vi "cps_serial_read.vi"(0 "serial in":refnum<visa-resource-name>, 8 "Range H":dbl, 9 "Range L":dbl=3.0) -> (1 "CK DATO":bool, 3 "Dato_ACK":u8, 4 "Allarme S":T1, 5 "AllarmeT":T1, 6 "CK Tot":bool, 7 "Allarme R":T1, 10 "Error Out":bool, 11 "Timeout":bool, 12 "Fase R":T3 {"Freq" format="%#.2g"; "Vout" format="%#.1f"; "Vset" format="%#.1f"}, 13 "Modo T":T2, 14 "Fase S":T3 {"Fase" format="%#.0f"; "Freq" format="%#.2g"; "Vout" format="%#.1f"; "Vset" format="%#.1f"}, 15 "Fase T":T3 {"Fase" format="%#.1f"; "Freq" format="%#.2g"; "Vout" format="%#.1f"; "Vset" format="%#.1f"}, 16 "DATI_RISP":u8[](array[numeric]), 17 "ACK":bool, 18 "Modo R":T2, 19 "Modo S":T2)   [LabVIEW 2019]
panel:
  in  "Timeout Limit":u32=3
  out "size(s)":i32
  out "Serial Read 3":string
  out "Bytes to Read":u32=10
  out "REPLY_PACKET":u8[](array[numeric])
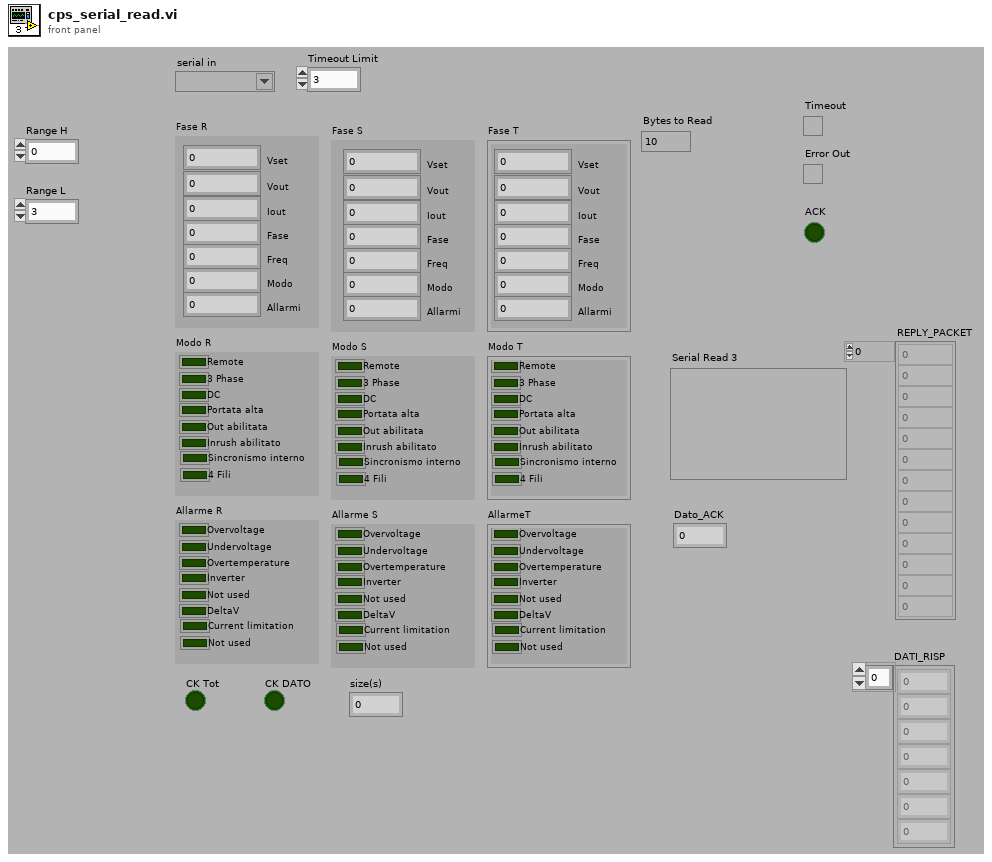
[diagram p1: front panel]
types:
  T1 = cluster{"Overvoltage":bool, "Undervoltage":bool, "Overtemperature":bool, "Inverter":bool, "Not used":bool, "DeltaV":bool, "Current limitation":bool, "Not used":bool}
  T2 = cluster{"Remote":bool, "3 Phase":bool, "DC":bool, "Portata alta":bool, "Out abilitata":bool, "Inrush abilitato":bool, "Sincronismo interno":bool, "4 Fili":bool}
  T3 = cluster{"Vset":dbl, "Vout":dbl, "Iout":dbl, "Freq":dbl, "Fase":dbl, "Modo":dbl, "Allarmi":dbl}
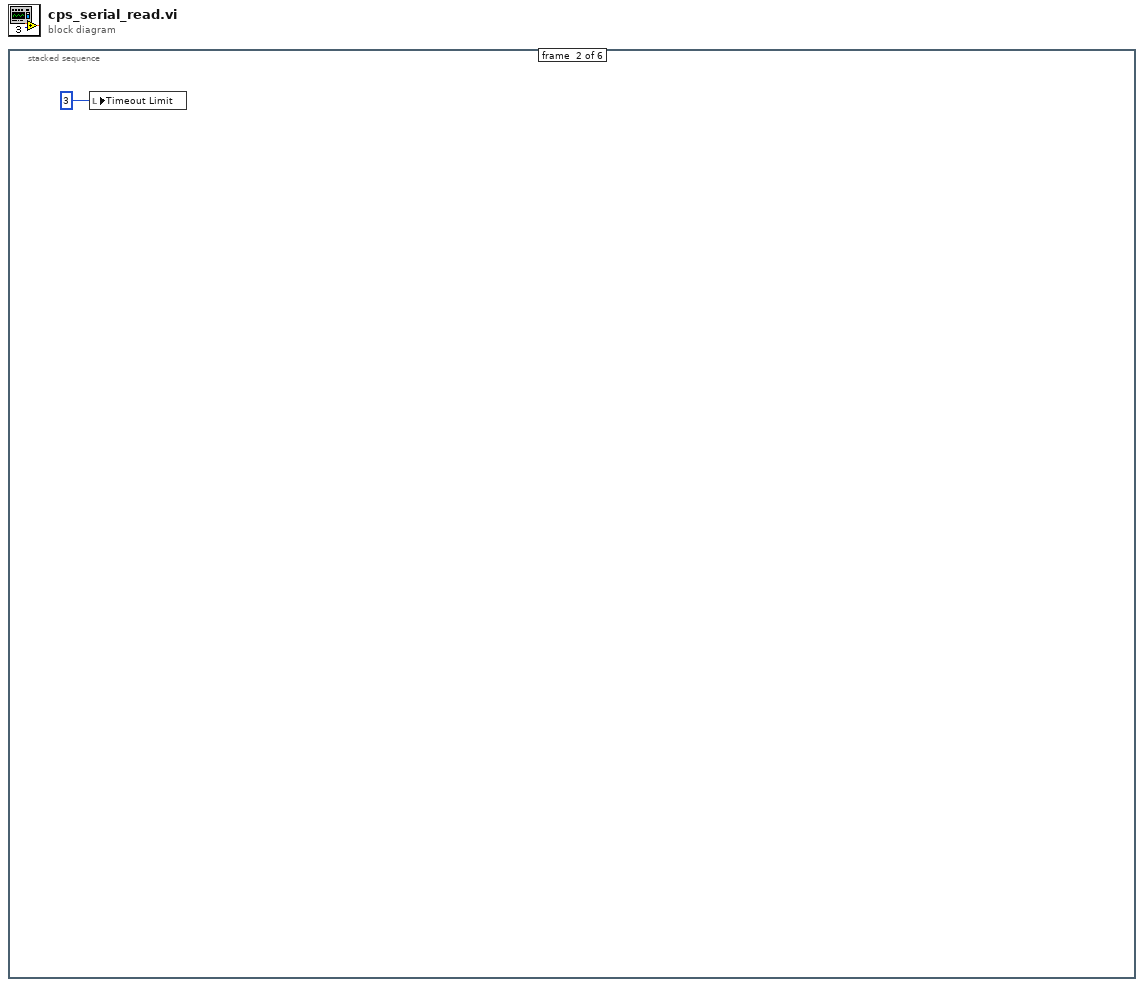
[diagram p0: block diagram]
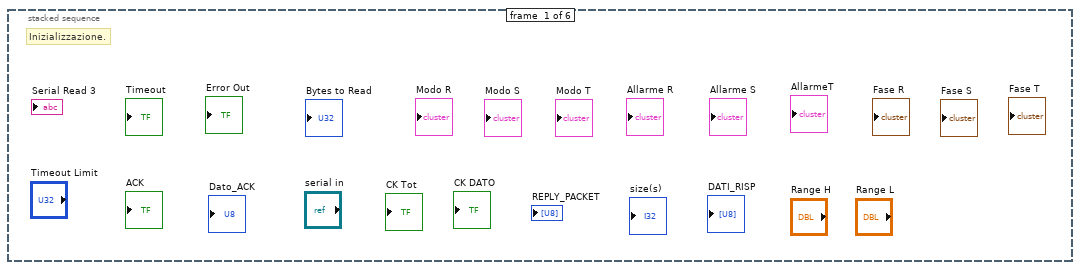
[diagram p2: hidden frame]
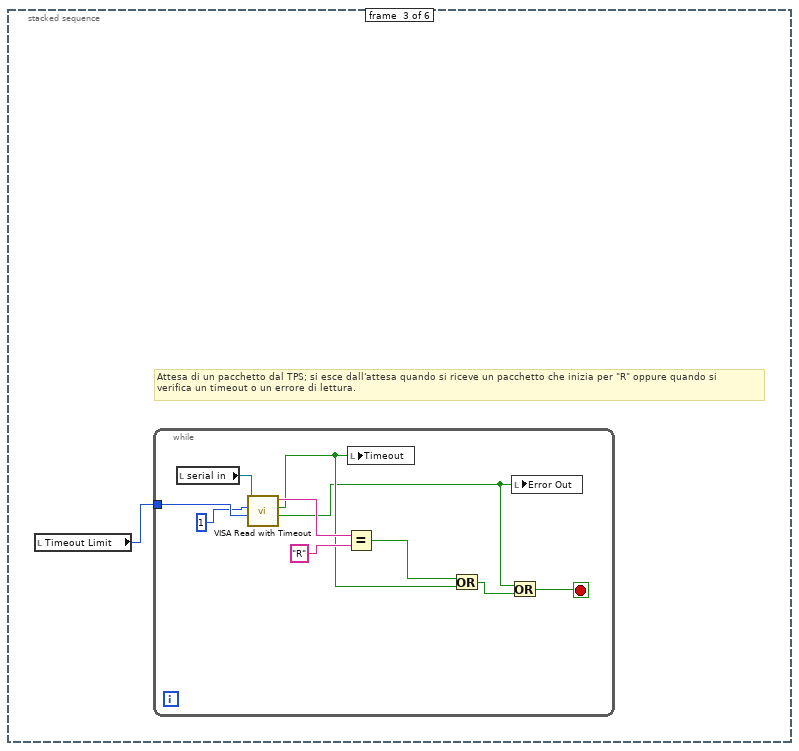
[diagram p3: hidden frame]
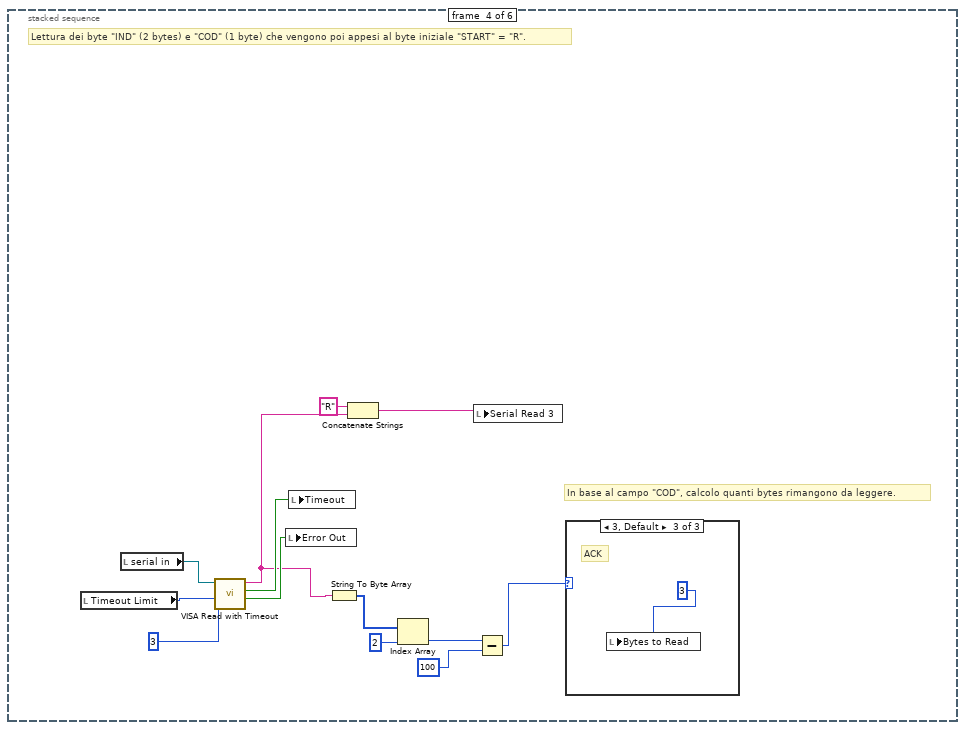
[diagram p4: hidden frame]
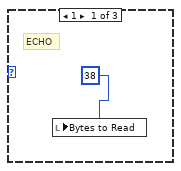
[diagram p5: hidden frame]
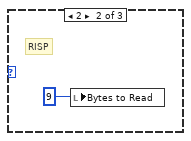
[diagram p6: hidden frame]
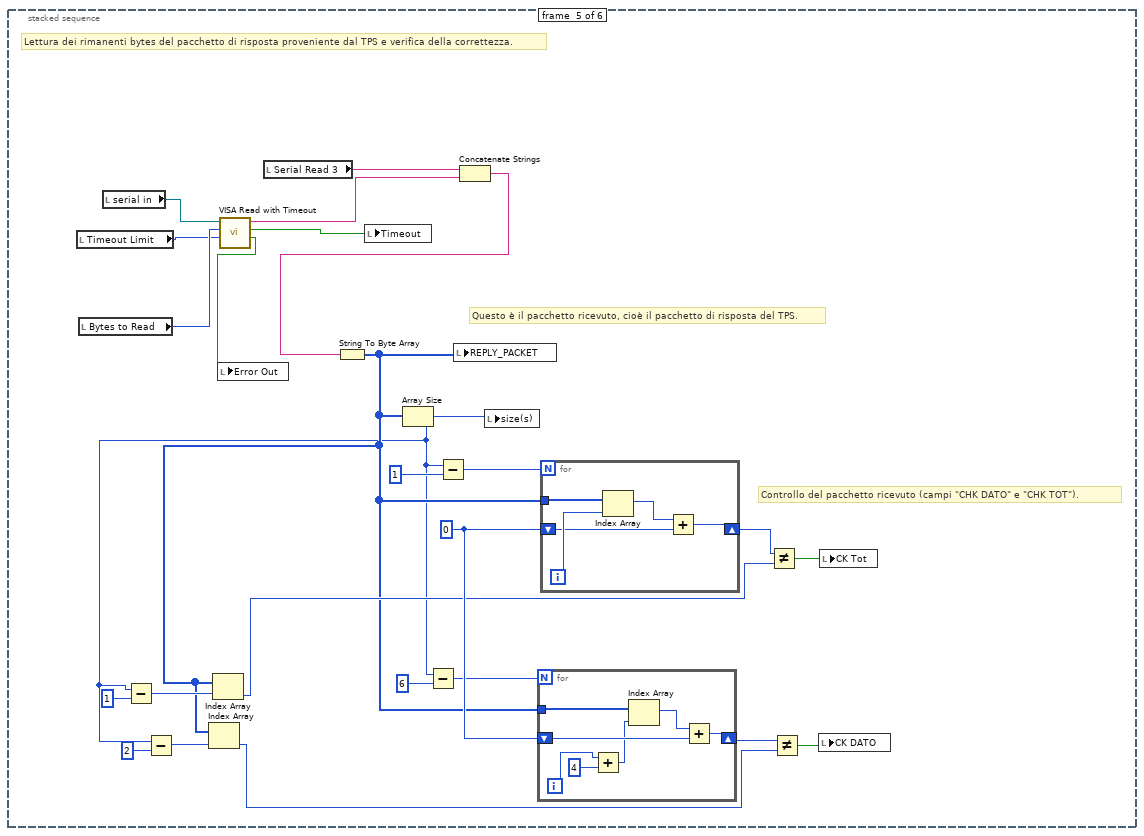
[diagram p7: hidden frame]
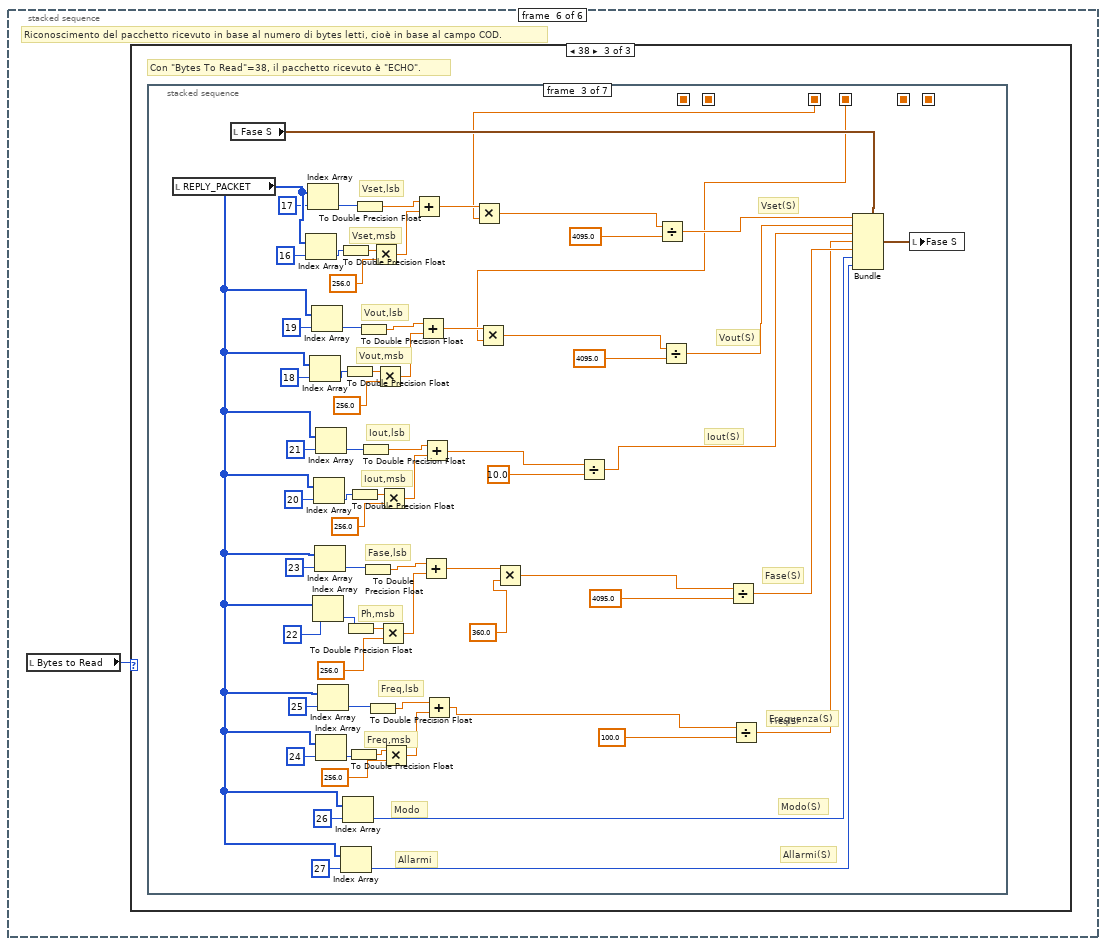
[diagram p8: hidden frame]
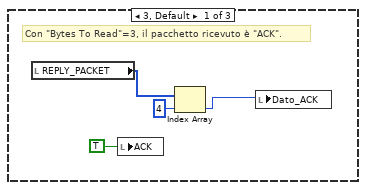
[diagram p9: hidden frame]
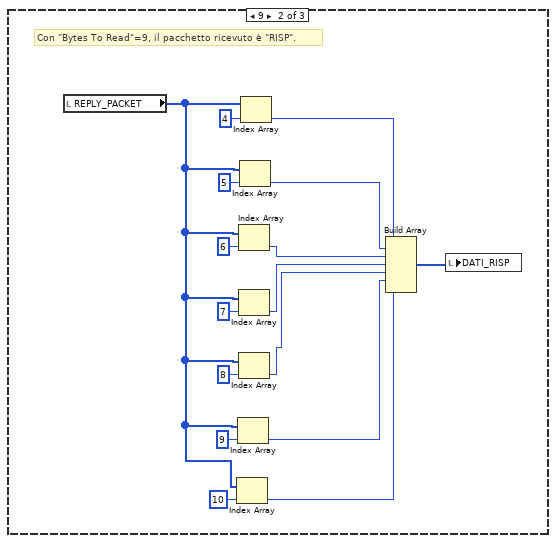
[diagram p10: hidden frame]
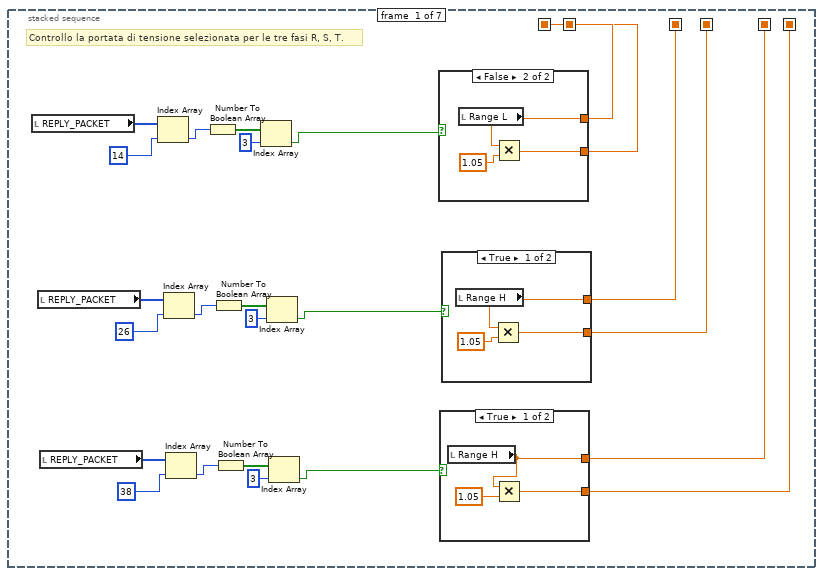
[diagram p11: hidden frame]
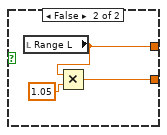
[diagram p12: hidden frame]
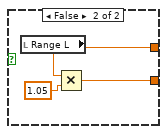
[diagram p13: hidden frame]
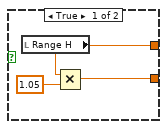
[diagram p14: hidden frame]
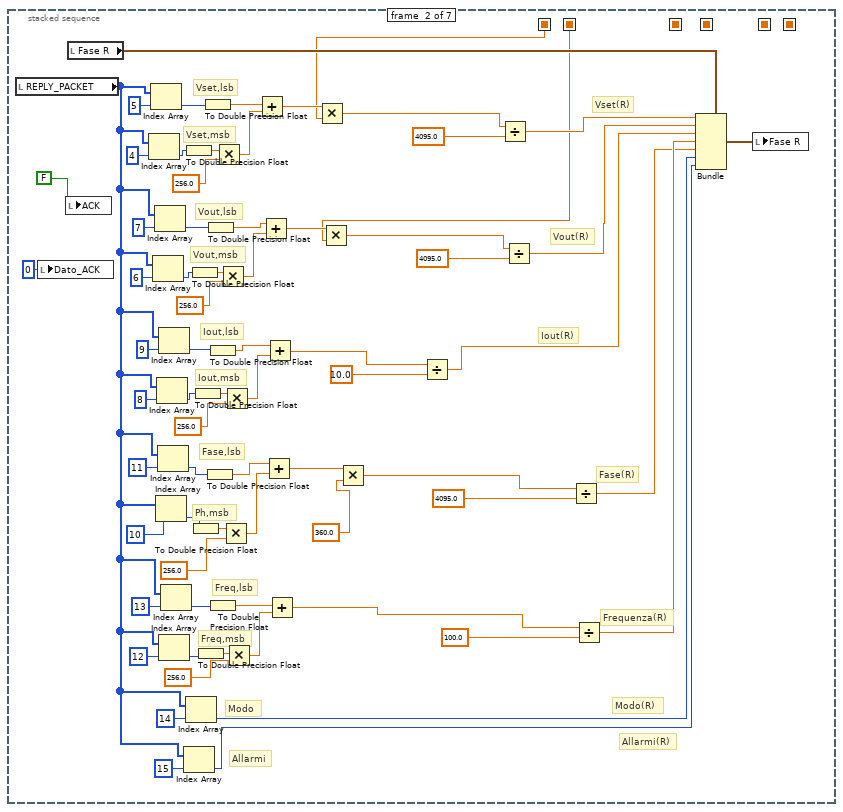
[diagram p15: hidden frame]
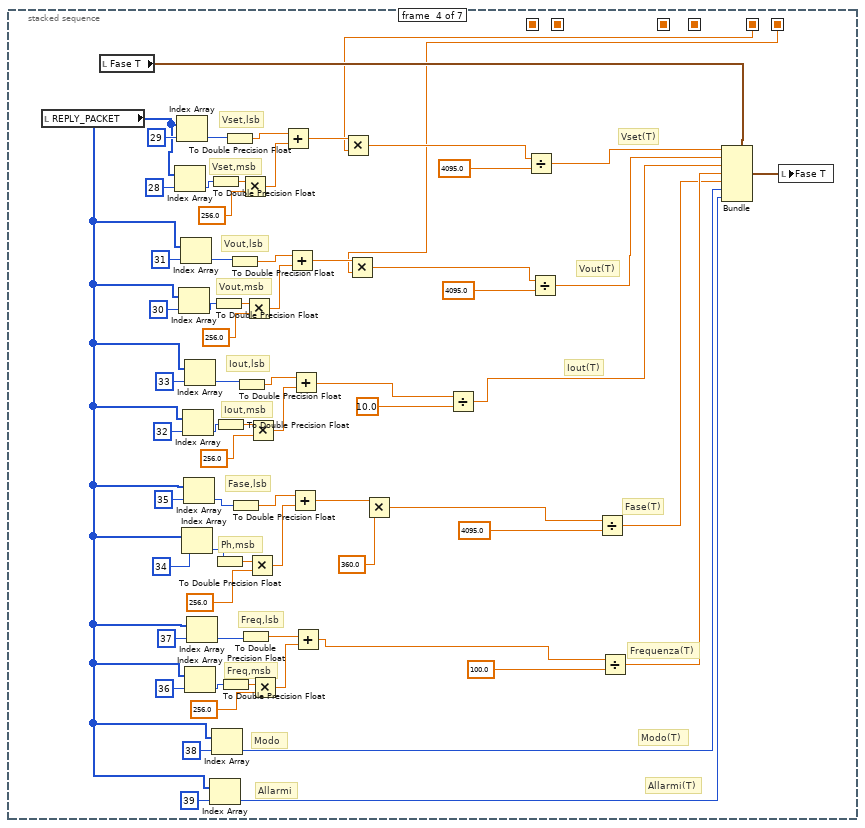
[diagram p16: hidden frame]
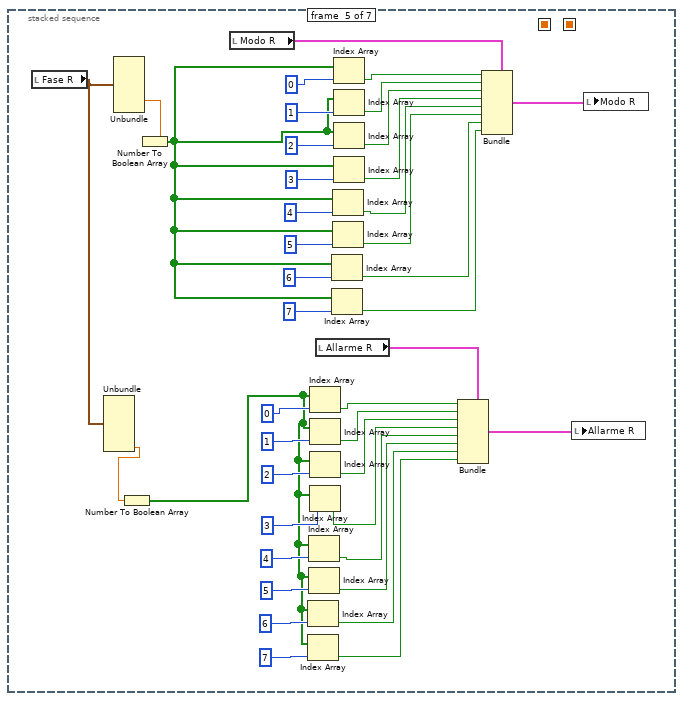
[diagram p17: hidden frame]
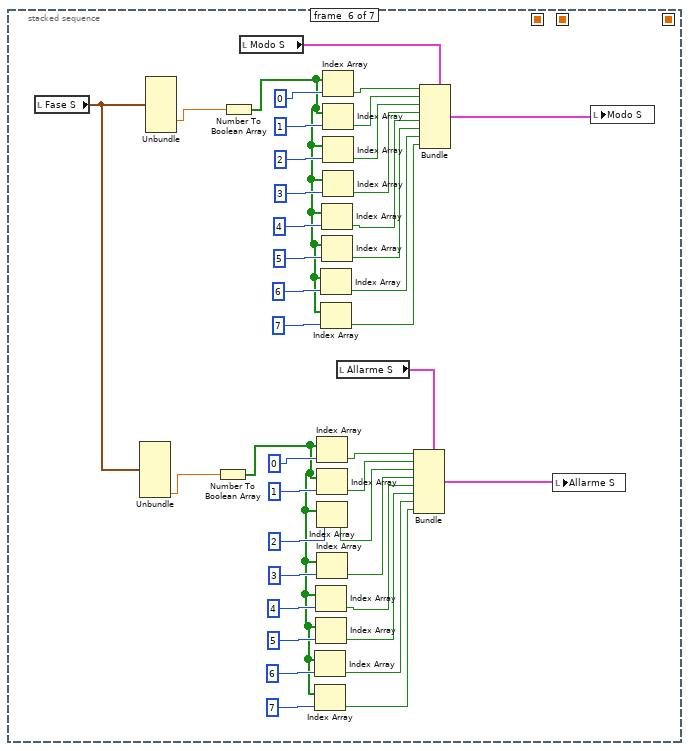
[diagram p18: hidden frame]
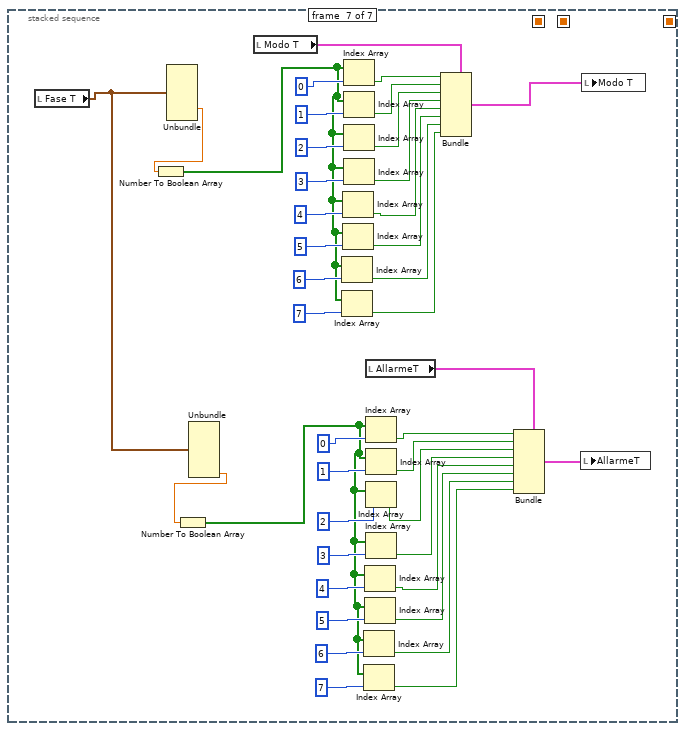
[diagram p19: hidden frame]
diagram:
  n1 = stacked-sequence {
    frame #0 {
      # "Inizializzazione."
    }
    frame #1 {
      n2 = local write "Timeout Limit"(u32 3 ("Timeout Limit")) -> ()
    }
    frame #2 {
      # "Attesa di un pacchetto dal TPS; si esce dall'attesa quando si riceve un pacchetto che inizia per \"R\" oppure quando si\nverifica un timeout o un errore di lettura."
      n3 = local read "Timeout Limit"() -> (w2:u32)
      n4 = while {
        tunnel: w2 -> [w12]
        stop <- w4 stop-if-true
        n5 = local read "serial in"() -> (w3:refnum<visa-resource-name>)
        n6 = call "VISA Read with Timeout.vi"("Timeout Limit"=w12, "Bytes to Read"=u32 1, "serial in"=w3) -> ("Error Out"=w5:bool, "Timeout"=w7:bool, "Serial Read"=w10:string)  [unwired: 1 in, 2 out]
        n7 = Equal?(x=w10, y="R") -> (x = y?=w8:bool)
        n8 = local write "Timeout"(w7) -> ()
        n9 = Or(x=w8, y=w7) -> (x .or. y?=w6:bool)
        n10 = Or(x=w5, y=w6) -> (x .or. y?=w4:bool)
        n11 = local write "Error Out"(w5) -> ()
      }
    }
    frame #3 {
      # "Lettura dei byte \"IND\" (2 bytes) e \"COD\" (1 byte) che vengono poi appesi al byte iniziale \"START\" = \"R\"."
      # "In base al campo \"COD\", calcolo quanti bytes rimangono da leggere."
      n12 = local read "Timeout Limit"() -> (w14:u32)
      n13 = local read "serial in"() -> (w13:refnum<visa-resource-name>)
      n14 = call "VISA Read with Timeout.vi"("Timeout Limit"=w14, "Bytes to Read"=u32 3, "serial in"=w13) -> ("Error Out"=w23:bool, "Timeout"=w24:bool, "Serial Read"=w20:string)  [unwired: 1 in, 2 out]
      n15 = local write "Error Out"(w23) -> ()
      n16 = local write "Timeout"(w24) -> ()
      n17 = String To Byte Array(string=w20) -> (unsigned byte array=w19:u8[])
      n18 = Concatenate Strings "Concatenate Strings"("R" ("string"), w20) -> (w21:string)
      n19 = Index Array "Index Array"(array=w19, index=2) -> (element=w17:u8)
      n20 = local write "Serial Read 3"(w21) -> ()
      n21 = Subtract(x=w17, y=u32 100 ("Bytes to Read")) -> (x-y=w16:u32)
      n22 = case shown="3, Default" w16 {
        frame 1 {
          # "ECHO"
          n23 = local write "Bytes to Read"(38 ("index")) -> ()
        }
        frame 2 {
          # "RISP"
          n24 = local write "Bytes to Read"(9 ("index")) -> ()
        }
        frame 3, Default {
          # "ACK"
          n25 = local write "Bytes to Read"(u32 3 ("Bytes to Read")) -> ()
        }
      }
    }
    frame #4 {
      w46 = u8 0
      # "Controllo del pacchetto ricevuto (campi \"CHK DATO\" e \"CHK TOT\")."
      # "Questo è il pacchetto ricevuto, cioè il pacchetto di risposta del TPS."
      # "Lettura dei rimanenti bytes del pacchetto di risposta proveniente dal TPS e verifica della correttezza."
      n26 = local read "Timeout Limit"() -> (w34:u32)
      n27 = local read "Bytes to Read"() -> (w43:u32)
      n28 = local read "serial in"() -> (w33:refnum<visa-resource-name>)
      n29 = call "VISA Read with Timeout.vi"("Timeout Limit"=w34, "Bytes to Read"=w43, "serial in"=w33) -> ("Error Out"=w53:bool, "Timeout"=w52:bool, "Serial Read"=w51:string)  [unwired: 1 in, 2 out]
      n30 = local write "Error Out"(w53) -> ()
      n31 = local read "Serial Read 3"() -> (w49:string)
      n32 = local write "Timeout"(w52) -> ()
      n33 = Concatenate Strings "Concatenate Strings"(w49, w51) -> (w50:string)
      n34 = String To Byte Array(string=w50) -> (unsigned byte array=w30:u8[])
      n35 = Array Size(array=w30) -> (size(s)=w29:i32)
      n36 = Subtract(x=w29, y=1) -> (x-y=w42:i32)
      n37 = Subtract(x=w29, y=2) -> (x-y=w41:i32)
      n38 = Index Array "Index Array"(array=w30, index=w41) -> (element=w35:u8)
      n39 = Index Array "Index Array"(array=w30, index=w42) -> (element=w37:u8)
      n40 = Subtract(x=w29, y=u8 6) -> (x-y=w45:i32)
      n41 = Subtract(x=w29, y=u8 1) -> (x-y=w47:i32)
      n42 = local write "REPLY_PACKET"(w30) -> ()
      n43 = local write "size(s)"(w29) -> ()
      n44 = for {
        N: w45 -> [_]
        tunnel: w30 -> [w60]
        shift-right: [w57] -> w36
        shift-left: w46 -> [w58]
        i -> [w55]
        n45 = Add(x=w55, y=u32 4) -> (x+y=w54:u32)
        n46 = Index Array(array=w60, index=w54) -> (element=w59:u8)
        n47 = Add(x=w59, y=w58) -> (x+y=w57:u8)
      }
      n48 = for {
        N: w47 -> [_]
        tunnel: w30 -> [w65]
        shift-right: [w61] -> w38
        shift-left: w46 -> [w62]
        i -> [w63]
        n49 = Index Array "Index Array"(array=w65, index=w63) -> (element=w64:u8)
        n50 = Add(x=w64, y=w62) -> (x+y=w61:u8)
      }
      n51 = Not Equal?(x=w38, y=w37) -> (x != y?=w32:bool)
      n52 = Not Equal?(x=w36, y=w35) -> (x != y?=w31:bool)
      n53 = local write "CK DATO"(w31) -> ()
      n54 = local write "CK Tot"(w32) -> ()
    }
    frame #5 {
      # "Riconoscimento del pacchetto ricevuto in base al numero di bytes letti, cioè in base al campo COD."
      n55 = local read "Bytes to Read"() -> (w66:u32)
      n56 = case shown="38" w66 {
        frame 3, Default {
          # "Con \"Bytes To Read\"=3, il pacchetto ricevuto è \"ACK\"."
          n57 = local read "REPLY_PACKET"() -> (w70:u8[])
          n58 = local write "ACK"(TRUE ("ACK")) -> ()
          n59 = Index Array "Index Array"(array=w70, index=4) -> (element=w67:u8)
          n60 = local write "Dato_ACK"(w67) -> ()
        }
        frame 9 {
          # "Con \"Bytes To Read\"=9, il pacchetto ricevuto è \"RISP\"."
          n61 = local read "REPLY_PACKET"() -> (w79:u8[])
          n62 = Index Array "Index Array"(array=w79, index=10) -> (element=w72:u8)
          n63 = Index Array "Index Array"(array=w79, index=9) -> (element=w73:u8)
          n64 = Index Array "Index Array"(array=w79, index=6) -> (element=w76:u8)
          n65 = Index Array "Index Array"(array=w79, index=7) -> (element=w75:u8)
          n66 = Index Array "Index Array"(array=w79, index=8) -> (element=w74:u8)
          n67 = Index Array "Index Array"(array=w79, index=5) -> (element=w77:u8)
          n68 = Index Array "Index Array"(array=w79, index=4) -> (element=w78:u8)
          n69 = Build Array(w78, w77, w76, w75, w74, w73, w72) -> (w71:u8[])
          n70 = local write "DATI_RISP"(w71) -> ()
        }
        frame 38 {
          # "Con \"Bytes To Read\"=38, il pacchetto ricevuto è \"ECHO\"."
          n71 = stacked-sequence {
            seq-local: [w110 _ _ _ _ _ _] -> [_ w150 _ _ _ _ _]
            seq-local: [w109 _ _ _ _ _ _] -> [_ w149 _ _ _ _ _]
            seq-local: [w108 _ _ _ _ _ _] -> [_ _ w220 _ _ _ _]
            seq-local: [w107 _ _ _ _ _ _] -> [_ _ w219 _ _ _ _]
            seq-local: [w106 _ _ _ _ _ _] -> [_ _ _ w288 _ _ _]
            seq-local: [w105 _ _ _ _ _ _] -> [_ _ _ w287 _ _ _]
            frame #0 {
              # "Controllo la portata di tensione selezionata per le tre fasi R, S, T."
              n72 = local read "REPLY_PACKET"() -> (w104:u8[])
              n73 = local read "REPLY_PACKET"() -> (w94:u8[])
              n74 = local read "REPLY_PACKET"() -> (w92:u8[])
              n75 = Index Array "Index Array"(array=w104, index=14) -> (element=w102:u8)
              n76 = Index Array "Index Array"(array=w94, index=26) -> (element=w96:u8)
              n77 = Index Array "Index Array"(array=w92, index=38) -> (element=w90:u8)
              n78 = Number To Boolean Array(number=w102) -> (Boolean array=w101:bool[])
              n79 = Number To Boolean Array(number=w96) -> (Boolean array=w97:bool[])
              n80 = Number To Boolean Array(number=w90) -> (Boolean array=w89:bool[])
              n81 = Index Array "Index Array"(array=w101, index=3) -> (element=w99:bool)
              n82 = Index Array "Index Array"(array=w97, index=3) -> (element=w93:bool)
              n83 = Index Array "Index Array"(array=w89, index=3) -> (element=w87:bool)
              n84 = case shown="False" w99 {
                tunnel: [w125 w127] -> w110
                tunnel: [w123 w128] -> w109
                frame True {
                  n85 = local read "Range H"() -> (w125:dbl)
                  n86 = Multiply(x=w125, y=1.05) -> (x*y=w123:dbl)
                }
                frame False {
                  n87 = local read "Range L"() -> (w127:dbl)
                  n88 = Multiply(x=w127, y=1.05) -> (x*y=w128:dbl)
                }
              }
              n89 = case shown="True" w87 {
                tunnel: [w112 w115] -> w106
                tunnel: [w113 w116] -> w105
                frame True {
                  n90 = local read "Range H"() -> (w112:dbl)
                  n91 = Multiply(x=w112, y=1.05) -> (x*y=w113:dbl)
                }
                frame False {
                  n92 = local read "Range L"() -> (w115:dbl)
                  n93 = Multiply(x=w115, y=1.05) -> (x*y=w116:dbl)
                }
              }
              n94 = case shown="True" w93 {
                tunnel: [w118 w121] -> w108
                tunnel: [w119 w122] -> w107
                frame True {
                  n95 = local read "Range H"() -> (w118:dbl)
                  n96 = Multiply(x=w118, y=1.05) -> (x*y=w119:dbl)
                }
                frame False {
                  n97 = local read "Range L"() -> (w121:dbl)
                  n98 = Multiply(x=w121, y=1.05) -> (x*y=w122:dbl)
                }
              }
            }
            frame #1 {
              # "Allarmi(R)"
              # "Modo(R)"
              # "Frequenza(R)"
              # "Fase(R)"
              # "Iout(R)"
              # "Vout(R)"
              # "Vset(R)"
              # "Allarmi"
              # "Modo"
              # "Freq,msb"
              # "Freq,lsb"
              # "Ph,msb"
              # "Fase,lsb"
              # "Iout,msb"
              # "Iout,lsb"
              # "Vout,msb"
              # "Vout,lsb"
              # "Vset,lsb"
              # "Vset,msb"
              n99 = local read "REPLY_PACKET"() -> (w153:u8[])
              n100 = local write "Dato_ACK"(u8 0 ("Dato_ACK")) -> ()
              n101 = local write "ACK"(FALSE ("ACK")) -> ()
              n102 = local read "Fase R"() -> (w184:T3)
              n103 = Index Array(array=w153, index=4) -> (element=w136:u8)
              n104 = Index Array "Index Array"(array=w153, index=5) -> (element=w148:u8)
              n105 = Index Array(array=w153, index=6) -> (element=w138:u8)
              n106 = Index Array(array=w153, index=7) -> (element=w146:u8)
              n107 = Index Array(array=w153, index=10) -> (element=w134:u8)
              n108 = Index Array(array=w153, index=8) -> (element=w140:u8)
              n109 = Index Array(array=w153, index=11) -> (element=w142:u8)
              n110 = Index Array(array=w153, index=9) -> (element=w144:u8)
              n111 = Index Array(array=w153, index=12) -> (element=w130:u8)
              n112 = Index Array(array=w153, index=13) -> (element=w132:u8)
              n113 = To Double Precision Float(number=w136) -> (double precision float=w135:dbl)
              n114 = Index Array(array=w153, index=15) -> (element=w155:u8)
              n115 = Index Array(array=w153, index=14) -> (element=w156:u8)
              n116 = To Double Precision Float(number=w138) -> (double precision float=w137:dbl)
              n117 = To Double Precision Float(number=w134) -> (double precision float=w133:dbl)
              n118 = To Double Precision Float(number=w140) -> (double precision float=w139:dbl)
              n119 = To Double Precision Float(number=w130) -> (double precision float=w129:dbl)
              n120 = To Double Precision Float(number=w148) -> (double precision float=w147:dbl)
              n121 = To Double Precision Float(number=w142) -> (double precision float=w141:dbl)
              n122 = To Double Precision Float(number=w146) -> (double precision float=w145:dbl)
              n123 = To Double Precision Float(number=w144) -> (double precision float=w143:dbl)
              n124 = To Double Precision Float(number=w132) -> (double precision float=w131:dbl)
              n125 = Multiply(x=w135, y=256.0) -> (x*y=w194:dbl)
              n126 = Multiply(x=w137, y=256.0) -> (x*y=w187:dbl)
              n127 = Multiply(x=w133, y=256.0) -> (x*y=w170:dbl)
              n128 = Multiply(x=w139, y=256.0) -> (x*y=w177:dbl)
              n129 = Multiply(x=w129, y=256.0) -> (x*y=w162:dbl)
              n130 = Add(x=w147, y=w194) -> (x+y=w193:dbl)
              n131 = Add(x=w145, y=w187) -> (x+y=w186:dbl)
              n132 = Add(x=w141, y=w170) -> (x+y=w166:dbl)
              n133 = Add(x=w143, y=w177) -> (x+y=w175:dbl)
              n134 = Add(x=w131, y=w162) -> (x+y=w154:dbl)
              n135 = Multiply(x=w193, y=w150) -> (x*y=w192:dbl)
              n136 = Multiply(x=w186, y=w149) -> (x*y=w185:dbl)
              n137 = Multiply(x=w166, y=360.0) -> (x*y=w167:dbl)
              n138 = Divide(x=w175, y=10.0) -> (x/y=w174:dbl)
              n139 = Divide(x=w192, y=4095.0) -> (x/y=w183:dbl)
              n140 = Divide(x=w185, y=4095.0) -> (x/y=w181:dbl)
              n141 = Divide(x=w167, y=4095.0) -> (x/y=w159:dbl)
              n142 = Divide(x=w154, y=100.0) -> (x/y=w160:dbl)
              n143 = Bundle "Bundle"(cluster=w184, "Vset"=w183, "Vout"=w181, "Iout"=w174, "Freq"=w160, "Fase"=w159, "Modo"=w156, "Allarmi"=w155) -> (w182:T3)
              n144 = local write "Fase R"(w182) -> ()
            }
            frame #2 {
              # "Allarmi(S)"
              # "Modo(S)"
              # "Frequenza(S)"
              # "Fase(S)"
              # "Iout(S)"
              # "Vout(S)"
              # "Vset(S)"
              # "Allarmi"
              # "Modo"
              # "Freq,msb"
              # "Freq,lsb"
              # "Ph,msb"
              # "Fase,lsb"
              # "Iout,msb"
              # "Iout,lsb"
              # "Vout,msb"
              # "Vout,lsb"
              # "Vset,lsb"
              # "Vset,msb"
              # "Freq(S)"
              n145 = local read "REPLY_PACKET"() -> (w263:u8[])
              n146 = local read "Fase S"() -> (w235:T3)
              n147 = Index Array(array=w263, index=16) -> (element=w216:u8)
              n148 = Index Array(array=w263, index=17) -> (element=w218:u8)
              n149 = Index Array(array=w263, index=18) -> (element=w212:u8)
              n150 = Index Array(array=w263, index=19) -> (element=w214:u8)
              n151 = Index Array(array=w263, index=22) -> (element=w204:u8)
              n152 = Index Array(array=w263, index=20) -> (element=w208:u8)
              n153 = Index Array(array=w263, index=23) -> (element=w206:u8)
              n154 = Index Array(array=w263, index=21) -> (element=w210:u8)
              n155 = Index Array(array=w263, index=24) -> (element=w200:u8)
              n156 = Index Array(array=w263, index=25) -> (element=w202:u8)
              n157 = To Double Precision Float(number=w216) -> (double precision float=w215:dbl)
              n158 = Index Array(array=w263, index=27) -> (element=w265:u8)
              n159 = Index Array(array=w263, index=26) -> (element=w264:u8)
              n160 = To Double Precision Float(number=w212) -> (double precision float=w211:dbl)
              n161 = To Double Precision Float(number=w204) -> (double precision float=w203:dbl)
              n162 = To Double Precision Float(number=w200) -> (double precision float=w199:dbl)
              n163 = To Double Precision Float(number=w208) -> (double precision float=w207:dbl)
              n164 = To Double Precision Float(number=w218) -> (double precision float=w217:dbl)
              n165 = To Double Precision Float(number=w214) -> (double precision float=w213:dbl)
              n166 = To Double Precision Float(number=w210) -> (double precision float=w209:dbl)
              n167 = To Double Precision Float(number=w206) -> (double precision float=w205:dbl)
              n168 = To Double Precision Float(number=w202) -> (double precision float=w201:dbl)
              n169 = Multiply(x=w215, y=256.0) -> (x*y=w225:dbl)
              n170 = Multiply(x=w211, y=256.0) -> (x*y=w232:dbl)
              n171 = Multiply(x=w203, y=256.0) -> (x*y=w249:dbl)
              n172 = Multiply(x=w207, y=256.0) -> (x*y=w242:dbl)
              n173 = Multiply(x=w199, y=256.0) -> (x*y=w257:dbl)
              n174 = Add(x=w217, y=w225) -> (x+y=w226:dbl)
              n175 = Add(x=w213, y=w232) -> (x+y=w233:dbl)
              n176 = Add(x=w205, y=w249) -> (x+y=w253:dbl)
              n177 = Add(x=w209, y=w242) -> (x+y=w244:dbl)
              n178 = Add(x=w201, y=w257) -> (x+y=w266:dbl)
              n179 = Multiply(x=w226, y=w220) -> (x*y=w227:dbl)
              n180 = Multiply(x=w233, y=w219) -> (x*y=w234:dbl)
              n181 = Multiply(x=w253, y=360.0) -> (x*y=w252:dbl)
              n182 = Divide(x=w244, y=10.0) -> (x/y=w245:dbl)
              n183 = Divide(x=w227, y=4095.0) -> (x/y=w236:dbl)
              n184 = Divide(x=w234, y=4095.0) -> (x/y=w238:dbl)
              n185 = Divide(x=w252, y=4095.0) -> (x/y=w260:dbl)
              n186 = Divide(x=w266, y=100.0) -> (x/y=w259:dbl)
              n187 = Bundle "Bundle"(cluster=w235, "Vset"=w236, "Vout"=w238, "Iout"=w245, "Freq"=w259, "Fase"=w260, "Modo"=w264, "Allarmi"=w265) -> (w237:T3)
              n188 = local write "Fase S"(w237) -> ()
            }
            frame #3 {
              # "Allarmi(T)"
              # "Modo(T)"
              # "Frequenza(T)"
              # "Fase(T)"
              # "Iout(T)"
              # "Vout(T)"
              # "Vset(T)"
              # "Allarmi"
              # "Modo"
              # "Freq,msb"
              # "Freq,lsb"
              # "Ph,msb"
              # "Fase,lsb"
              # "Iout,msb"
              # "Iout,lsb"
              # "Vout,msb"
              # "Vout,lsb"
              # "Vset,lsb"
              # "Vset,msb"
              n189 = local read "REPLY_PACKET"() -> (w292:u8[])
              n190 = local read "Fase T"() -> (w320:T3)
              n191 = Index Array(array=w292, index=28) -> (element=w284:u8)
              n192 = Index Array(array=w292, index=29) -> (element=w286:u8)
              n193 = Index Array(array=w292, index=30) -> (element=w280:u8)
              n194 = Index Array(array=w292, index=31) -> (element=w282:u8)
              n195 = Index Array(array=w292, index=34) -> (element=w272:u8)
              n196 = Index Array(array=w292, index=32) -> (element=w276:u8)
              n197 = Index Array(array=w292, index=35) -> (element=w274:u8)
              n198 = Index Array(array=w292, index=33) -> (element=w278:u8)
              n199 = Index Array(array=w292, index=36) -> (element=w268:u8)
              n200 = Index Array(array=w292, index=37) -> (element=w270:u8)
              n201 = Index Array(array=w292, index=39) -> (element=w290:u8)
              n202 = To Double Precision Float(number=w284) -> (double precision float=w283:dbl)
              n203 = Index Array(array=w292, index=38) -> (element=w291:u8)
              n204 = To Double Precision Float(number=w280) -> (double precision float=w279:dbl)
              n205 = To Double Precision Float(number=w272) -> (double precision float=w271:dbl)
              n206 = To Double Precision Float(number=w276) -> (double precision float=w275:dbl)
              n207 = To Double Precision Float(number=w268) -> (double precision float=w267:dbl)
              n208 = To Double Precision Float(number=w286) -> (double precision float=w285:dbl)
              n209 = To Double Precision Float(number=w282) -> (double precision float=w281:dbl)
              n210 = To Double Precision Float(number=w274) -> (double precision float=w273:dbl)
              n211 = To Double Precision Float(number=w278) -> (double precision float=w277:dbl)
              n212 = Multiply(x=w283, y=256.0) -> (x*y=w330:dbl)
              n213 = To Double Precision Float(number=w270) -> (double precision float=w269:dbl)
              n214 = Multiply(x=w279, y=256.0) -> (x*y=w323:dbl)
              n215 = Multiply(x=w271, y=256.0) -> (x*y=w306:dbl)
              n216 = Multiply(x=w275, y=256.0) -> (x*y=w313:dbl)
              n217 = Multiply(x=w267, y=256.0) -> (x*y=w298:dbl)
              n218 = Add(x=w285, y=w330) -> (x+y=w329:dbl)
              n219 = Add(x=w281, y=w323) -> (x+y=w322:dbl)
              n220 = Add(x=w273, y=w306) -> (x+y=w302:dbl)
              n221 = Add(x=w277, y=w313) -> (x+y=w311:dbl)
              n222 = Add(x=w269, y=w298) -> (x+y=w289:dbl)
              n223 = Multiply(x=w329, y=w288) -> (x*y=w328:dbl)
              n224 = Multiply(x=w322, y=w287) -> (x*y=w321:dbl)
              n225 = Multiply(x=w302, y=360.0) -> (x*y=w303:dbl)
              n226 = Divide(x=w311, y=10.0) -> (x/y=w310:dbl)
              n227 = Divide(x=w328, y=4095.0) -> (x/y=w319:dbl)
              n228 = Divide(x=w321, y=4095.0) -> (x/y=w317:dbl)
              n229 = Divide(x=w303, y=4095.0) -> (x/y=w295:dbl)
              n230 = Divide(x=w289, y=100.0) -> (x/y=w296:dbl)
              n231 = Bundle "Bundle"(cluster=w320, "Vset"=w319, "Vout"=w317, "Iout"=w310, "Freq"=w296, "Fase"=w295, "Modo"=w291, "Allarmi"=w290) -> (w318:T3)
              n232 = local write "Fase T"(w318) -> ()
            }
            frame #4 {
              n233 = local read "Fase R"() -> (w339:T3)
              n234 = Unbundle "Unbundle"(w339) -> ("Allarmi"=w335:dbl)  [unwired: 6 out]
              n235 = Unbundle "Unbundle"(w339) -> ("Modo"=w336:dbl)  [unwired: 6 out]
              n236 = Number To Boolean Array(number=w335) -> (Boolean array=w348:bool[])
              n237 = Number To Boolean Array(number=w336) -> (Boolean array=w366:bool[])
              n238 = local read "Modo R"() -> (w375:T2)
              n239 = Index Array(array=w348, index=6) -> (element=w345:bool)
              n240 = Index Array(array=w348, index=7) -> (element=w346:bool)
              n241 = Index Array(array=w348, index=4) -> (element=w343:bool)
              n242 = Index Array(array=w348, index=5) -> (element=w344:bool)
              n243 = Index Array "Index Array"(array=w348, index=0) -> (element=w347:bool)
              n244 = Index Array(array=w348, index=1) -> (element=w340:bool)
              n245 = Index Array(array=w348, index=2) -> (element=w341:bool)
              n246 = Index Array(array=w348, index=3) -> (element=w342:bool)
              n247 = local read "Allarme R"() -> (w338:T1)
              n248 = Index Array(array=w366, index=6) -> (element=w363:bool)
              n249 = Index Array(array=w366, index=7) -> (element=w364:bool)
              n250 = Index Array(array=w366, index=4) -> (element=w361:bool)
              n251 = Index Array(array=w366, index=5) -> (element=w362:bool)
              n252 = Index Array "Index Array"(array=w366, index=0) -> (element=w365:bool)
              n253 = Index Array(array=w366, index=1) -> (element=w358:bool)
              n254 = Index Array(array=w366, index=2) -> (element=w359:bool)
              n255 = Index Array(array=w366, index=3) -> (element=w360:bool)
              n256 = Bundle(cluster=w338, "Overvoltage"=w347, "Undervoltage"=w340, "Overtemperature"=w341, "Inverter"=w342, "Not used"=w343, "DeltaV"=w344, "Current limitation"=w345, "Not used"=w346) -> (w337:T1)
              n257 = Bundle "Bundle"(cluster=w375, "Remote"=w365, "3 Phase"=w358, "DC"=w359, "Portata alta"=w360, "Out abilitata"=w361, "Inrush abilitato"=w362, "Sincronismo interno"=w363, "4 Fili"=w364) -> (w357:T2)
              n258 = local write "Allarme R"(w337) -> ()
              n259 = local write "Modo R"(w357) -> ()
            }
            frame #5 {
              n260 = local read "Fase S"() -> (w380:T3)
              n261 = Unbundle(w380) -> ("Allarmi"=w376:dbl)  [unwired: 6 out]
              n262 = Unbundle "Unbundle"(w380) -> ("Modo"=w377:dbl)  [unwired: 6 out]
              n263 = Number To Boolean Array(number=w376) -> (Boolean array=w389:bool[])
              n264 = Number To Boolean Array(number=w377) -> (Boolean array=w408:bool[])
              n265 = local read "Modo S"() -> (w399:T2)
              n266 = Index Array(array=w389, index=6) -> (element=w386:bool)
              n267 = Index Array(array=w389, index=7) -> (element=w387:bool)
              n268 = Index Array(array=w389, index=4) -> (element=w384:bool)
              n269 = Index Array(array=w389, index=5) -> (element=w385:bool)
              n270 = Index Array "Index Array"(array=w389, index=0) -> (element=w388:bool)
              n271 = Index Array(array=w389, index=1) -> (element=w381:bool)
              n272 = Index Array(array=w389, index=2) -> (element=w382:bool)
              n273 = Index Array(array=w389, index=3) -> (element=w383:bool)
              n274 = Index Array(array=w408, index=6) -> (element=w405:bool)
              n275 = Index Array(array=w408, index=7) -> (element=w406:bool)
              n276 = Index Array(array=w408, index=4) -> (element=w403:bool)
              n277 = Index Array(array=w408, index=5) -> (element=w404:bool)
              n278 = Index Array "Index Array"(array=w408, index=0) -> (element=w407:bool)
              n279 = Index Array(array=w408, index=1) -> (element=w400:bool)
              n280 = Index Array(array=w408, index=2) -> (element=w401:bool)
              n281 = Index Array(array=w408, index=3) -> (element=w402:bool)
              n282 = local read "Allarme S"() -> (w379:T1)
              n283 = Bundle(cluster=w379, "Overvoltage"=w388, "Undervoltage"=w381, "Overtemperature"=w382, "Inverter"=w383, "Not used"=w384, "DeltaV"=w385, "Current limitation"=w386, "Not used"=w387) -> (w378:T1)
              n284 = Bundle(cluster=w399, "Remote"=w407, "3 Phase"=w400, "DC"=w401, "Portata alta"=w402, "Out abilitata"=w403, "Inrush abilitato"=w404, "Sincronismo interno"=w405, "4 Fili"=w406) -> (w398:T2)
              n285 = local write "Allarme S"(w378) -> ()
              n286 = local write "Modo S"(w398) -> ()
            }
            frame #6 {
              n287 = local read "Fase T"() -> (w419:T3)
              n288 = Unbundle "Unbundle"(w419) -> ("Modo"=w418:dbl)  [unwired: 6 out]
              n289 = Number To Boolean Array(number=w418) -> (Boolean array=w449:bool[])
              n290 = Unbundle "Unbundle"(w419) -> ("Allarmi"=w417:dbl)  [unwired: 6 out]
              n291 = Number To Boolean Array(number=w417) -> (Boolean array=w430:bool[])
              n292 = local read "Modo T"() -> (w440:T2)
              n293 = Index Array(array=w449, index=6) -> (element=w446:bool)
              n294 = Index Array(array=w449, index=7) -> (element=w447:bool)
              n295 = Index Array(array=w449, index=4) -> (element=w444:bool)
              n296 = Index Array(array=w449, index=5) -> (element=w445:bool)
              n297 = Index Array "Index Array"(array=w449, index=0) -> (element=w448:bool)
              n298 = Index Array(array=w449, index=1) -> (element=w441:bool)
              n299 = Index Array(array=w449, index=2) -> (element=w442:bool)
              n300 = Index Array(array=w449, index=3) -> (element=w443:bool)
              n301 = Index Array(array=w430, index=6) -> (element=w427:bool)
              n302 = Index Array(array=w430, index=7) -> (element=w428:bool)
              n303 = Index Array(array=w430, index=4) -> (element=w425:bool)
              n304 = Index Array(array=w430, index=5) -> (element=w426:bool)
              n305 = local read "AllarmeT"() -> (w421:T1)
              n306 = Index Array "Index Array"(array=w430, index=0) -> (element=w429:bool)
              n307 = Index Array(array=w430, index=1) -> (element=w422:bool)
              n308 = Index Array(array=w430, index=2) -> (element=w423:bool)
              n309 = Index Array(array=w430, index=3) -> (element=w424:bool)
              n310 = Bundle "Bundle"(cluster=w440, "Remote"=w448, "3 Phase"=w441, "DC"=w442, "Portata alta"=w443, "Out abilitata"=w444, "Inrush abilitato"=w445, "Sincronismo interno"=w446, "4 Fili"=w447) -> (w439:T2)
              n311 = Bundle "Bundle"(cluster=w421, "Overvoltage"=w429, "Undervoltage"=w422, "Overtemperature"=w423, "Inverter"=w424, "Not used"=w425, "DeltaV"=w426, "Current limitation"=w427, "Not used"=w428) -> (w420:T1)
              n312 = local write "AllarmeT"(w420) -> ()
              n313 = local write "Modo T"(w439) -> ()
            }
          }
        }
      }
    }
  }
